vi "data_read.vi"() -> ()   [LabVIEW 2020]
uses:
  <vilib>/Utility/file.llb/Read Delimited Spreadsheet (DBL).vi
panel:
  out "XY Graph":cluster{"all rows":dbl[], "all rows":dbl[]}[](graph)
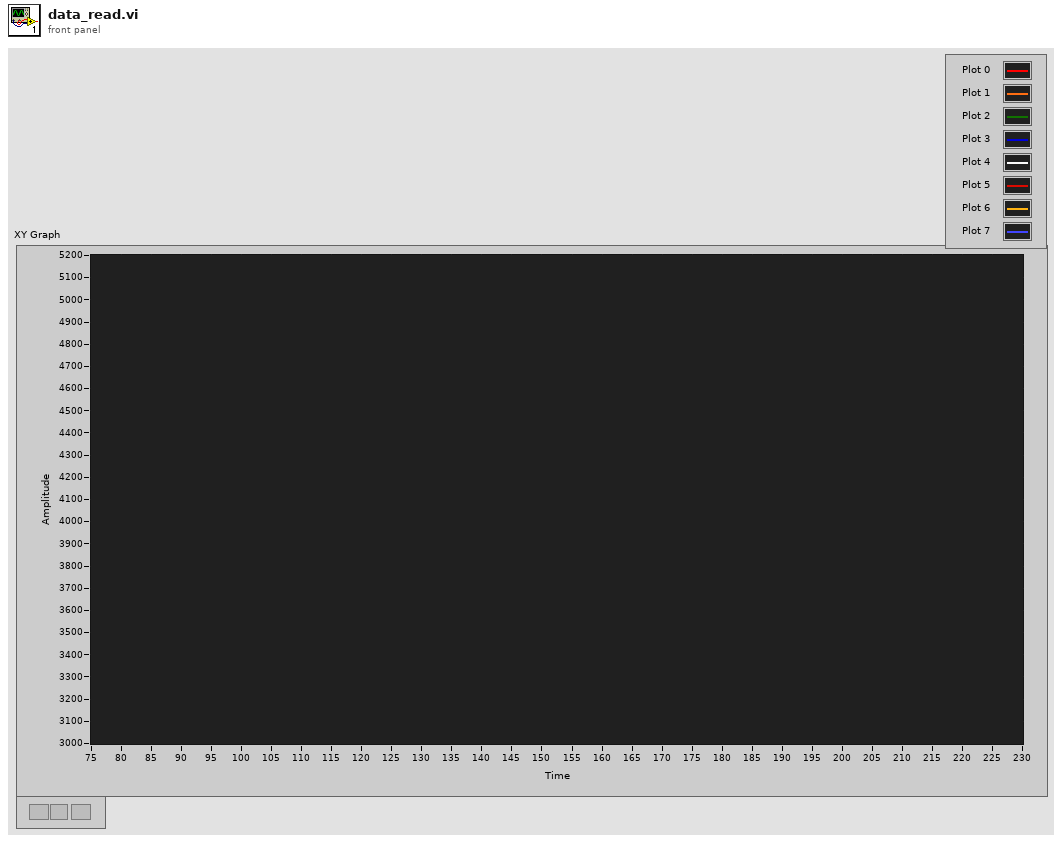
[diagram p1: front panel]
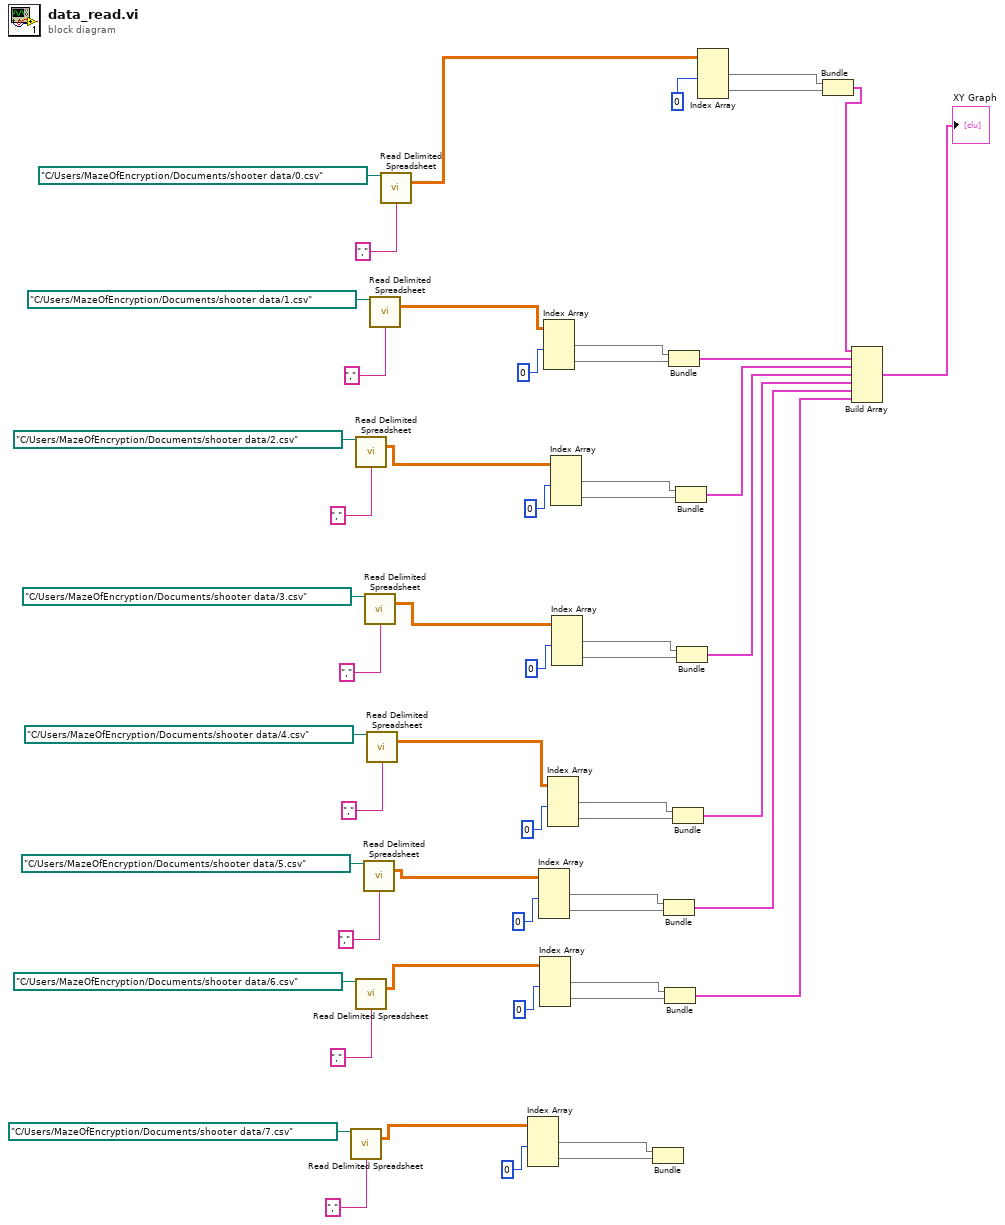
[diagram p0: block diagram]
diagram:
  n1 = call-poly <vilib>:"Read Delimited Spreadsheet.vi"("file path (dialog if empty)"=path "C:/Users/MazeOfEncryption/Documents/shooter data/7.csv", "delimiter (\\t)"="," ("delimiter (\\t)")) -> ("all rows"=w14:dbl[][])  [unwired: 8 in, 5 out]
  n2 = call-poly <vilib>:"Read Delimited Spreadsheet.vi"("file path (dialog if empty)"=path "C:/Users/MazeOfEncryption/Documents/shooter data/2.csv", "delimiter (\\t)"="," ("delimiter (\\t)")) -> ("all rows"=w9:dbl[][])  [unwired: 8 in, 5 out]
  n3 = call-poly <vilib>:"Read Delimited Spreadsheet.vi"("file path (dialog if empty)"=path "C:/Users/MazeOfEncryption/Documents/shooter data/6.csv", "delimiter (\\t)"="," ("delimiter (\\t)")) -> ("all rows"=w13:dbl[][])  [unwired: 8 in, 5 out]
  n4 = call-poly <vilib>:"Read Delimited Spreadsheet.vi"("file path (dialog if empty)"=path "C:/Users/MazeOfEncryption/Documents/shooter data/5.csv", "delimiter (\\t)"="," ("delimiter (\\t)")) -> ("all rows"=w12:dbl[][])  [unwired: 8 in, 5 out]
  n5 = call-poly <vilib>:"Read Delimited Spreadsheet.vi"("file path (dialog if empty)"=path "C:/Users/MazeOfEncryption/Documents/shooter data/3.csv", "delimiter (\\t)"="," ("delimiter (\\t)")) -> ("all rows"=w10:dbl[][])  [unwired: 8 in, 5 out]
  n6 = call-poly <vilib>:"Read Delimited Spreadsheet.vi"("file path (dialog if empty)"=path "C:/Users/MazeOfEncryption/Documents/shooter data/4.csv", "delimiter (\\t)"="," ("delimiter (\\t)")) -> ("all rows"=w11:dbl[][])  [unwired: 8 in, 5 out]
  n7 = call-poly <vilib>:"Read Delimited Spreadsheet.vi"("file path (dialog if empty)"=path "C:/Users/MazeOfEncryption/Documents/shooter data/1.csv", "delimiter (\\t)"="," ("delimiter (\\t)")) -> ("all rows"=w33:dbl[][])  [unwired: 8 in, 5 out]
  n8 = call-poly <vilib>:"Read Delimited Spreadsheet.vi"("file path (dialog if empty)"=path "C:/Users/MazeOfEncryption/Documents/shooter data/0.csv", "delimiter (\\t)"="," ("delimiter (\\t)")) -> ("all rows"=w54:dbl[][])  [unwired: 8 in, 5 out]
  n9 = Index Array(array=w14, index (col) #1=0 ("disabled index (col)")) -> (element #1=w16:dbl[], element #2=w17:dbl[])  [unwired: 3 in]
  n10 = Index Array(array=w12, index (col) #1=0 ("disabled index (col)")) -> (element #1=w22:dbl[], element #2=w23:dbl[])  [unwired: 3 in]
  n11 = Index Array(array=w13, index (col) #1=0 ("disabled index (col)")) -> (element #1=w19:dbl[], element #2=w18:dbl[])  [unwired: 3 in]
  n12 = Index Array(array=w33, index (col) #1=0 ("disabled index (col)")) -> (element #1=w35:dbl[], element #2=w36:dbl[])  [unwired: 3 in]
  n13 = Index Array(array=w11, index (col) #1=0 ("disabled index (col)")) -> (element #1=w25:dbl[], element #2=w24:dbl[])  [unwired: 3 in]
  n14 = Index Array(array=w9, index (col) #1=0 ("disabled index (col)")) -> (element #1=w31:dbl[], element #2=w30:dbl[])  [unwired: 3 in]
  n15 = Index Array(array=w10, index (col) #1=0 ("disabled index (col)")) -> (element #1=w28:dbl[], element #2=w29:dbl[])  [unwired: 3 in]
  n16 = Bundle("all rows"=w16, "all rows"=w17) -> ()  [unwired: 1 in, 1 out]
  n17 = Bundle("all rows"=w22, "all rows"=w23) -> (w4:cluster{"all rows":dbl[], "all rows":dbl[]})  [unwired: 1 in]
  n18 = Bundle("all rows"=w19, "all rows"=w18) -> (w3:cluster{"all rows":dbl[], "all rows":dbl[]})  [unwired: 1 in]
  n19 = Bundle("all rows"=w35, "all rows"=w36) -> (w8:cluster{"all rows":dbl[], "all rows":dbl[]})  [unwired: 1 in]
  n20 = Bundle("all rows"=w25, "all rows"=w24) -> (w5:cluster{"all rows":dbl[], "all rows":dbl[]})  [unwired: 1 in]
  n21 = Bundle("all rows"=w31, "all rows"=w30) -> (w7:cluster{"all rows":dbl[], "all rows":dbl[]})  [unwired: 1 in]
  n22 = Bundle("all rows"=w28, "all rows"=w29) -> (w6:cluster{"all rows":dbl[], "all rows":dbl[]})  [unwired: 1 in]
  n23 = Index Array(array=w54, index (col) #1=0 ("disabled index (col)")) -> (element #1=w53:dbl[], element #2=w52:dbl[])  [unwired: 3 in]
  n24 = Bundle("all rows"=w53, "all rows"=w52) -> (w2:cluster{"all rows":dbl[], "all rows":dbl[]})  [unwired: 1 in]
  n25 = Build Array(w2, w8, w7, w6, w5, w4, w3) -> (→"XY Graph":cluster{"all rows":dbl[], "all rows":dbl[]}[])
